vi "Initialize P40.vi"(8 "error in (no error)":errorcluster, 11 "SSI P40 Settings In":T1={"VISA resource name"="", "Simulated?"=TRUE}) -> (0 "error out":errorcluster, 1 "Initialized":bool, 2 "No Pump Connected":bool, 3 "SSI P40 Settings Out":T1={"VISA resource name"="", "Simulated?"=TRUE})   [LabVIEW 2021, in "SSI P40 Pump.lvlib"]
uses:
  SSI P40 Pump.lvlib
  SSI P40 Settings Cluster.ctl
  <vilib>/Instr/_visa.llb/VISA Configure Serial Port (Instr).vi
  <vilib>/regexp/Match Regular Expression.xnode
panel:
  out "read buffer 2":string
  out "read buffer":string
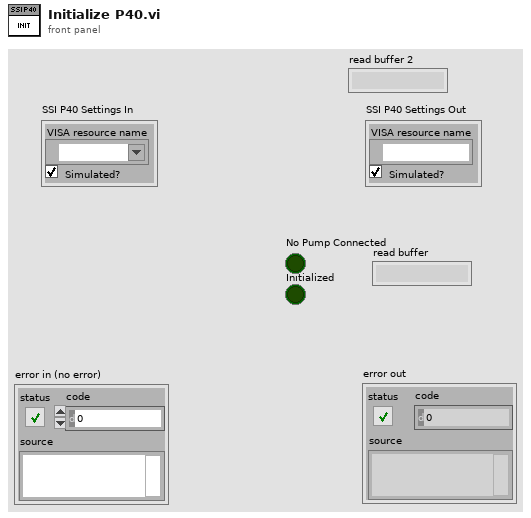
[diagram p1: front panel]
types:
  T1 = typedef "SSI P40 Pump.lvlib/SSI P40 Settings Cluster.ctl" = cluster{"VISA resource name":refnum<visa-resource-name>, "Simulated?":bool}
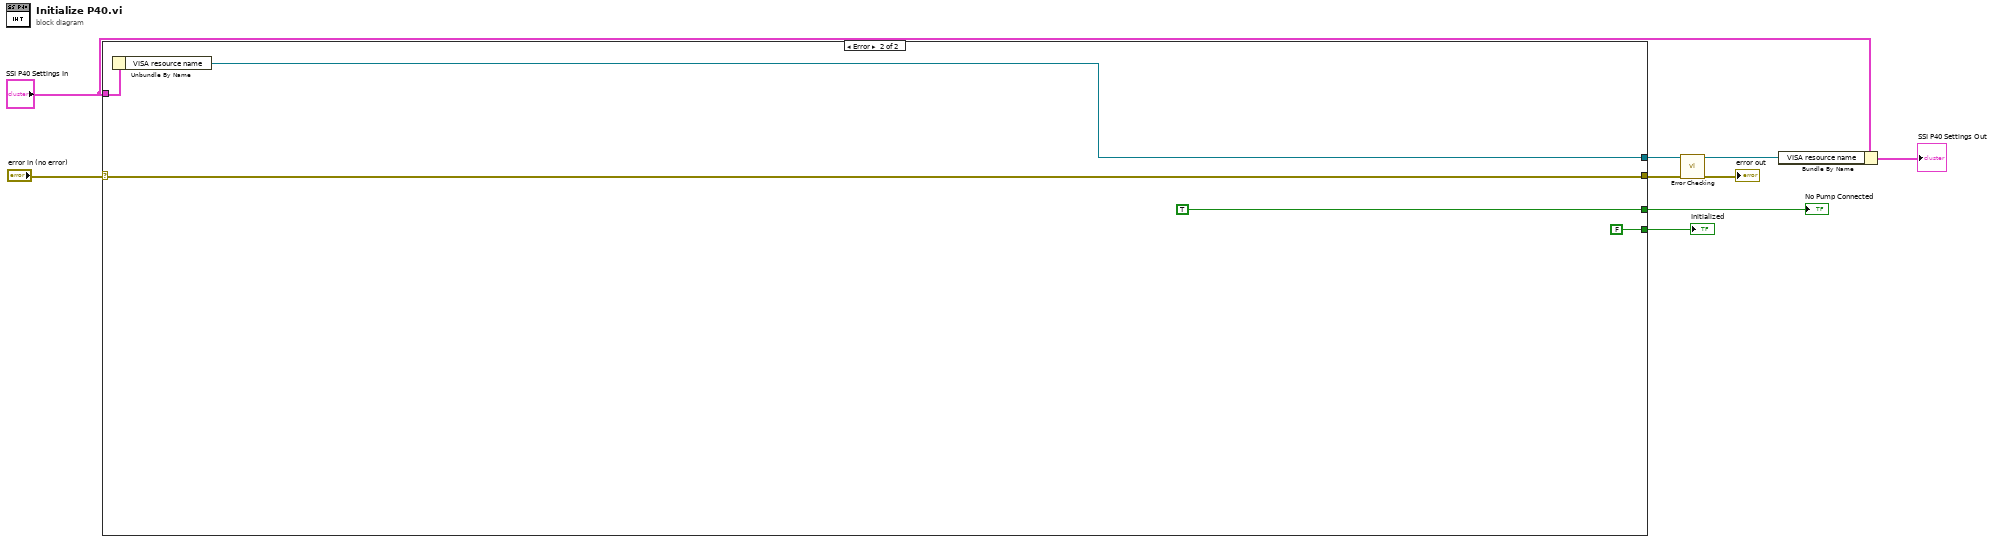
[diagram p0: block diagram]
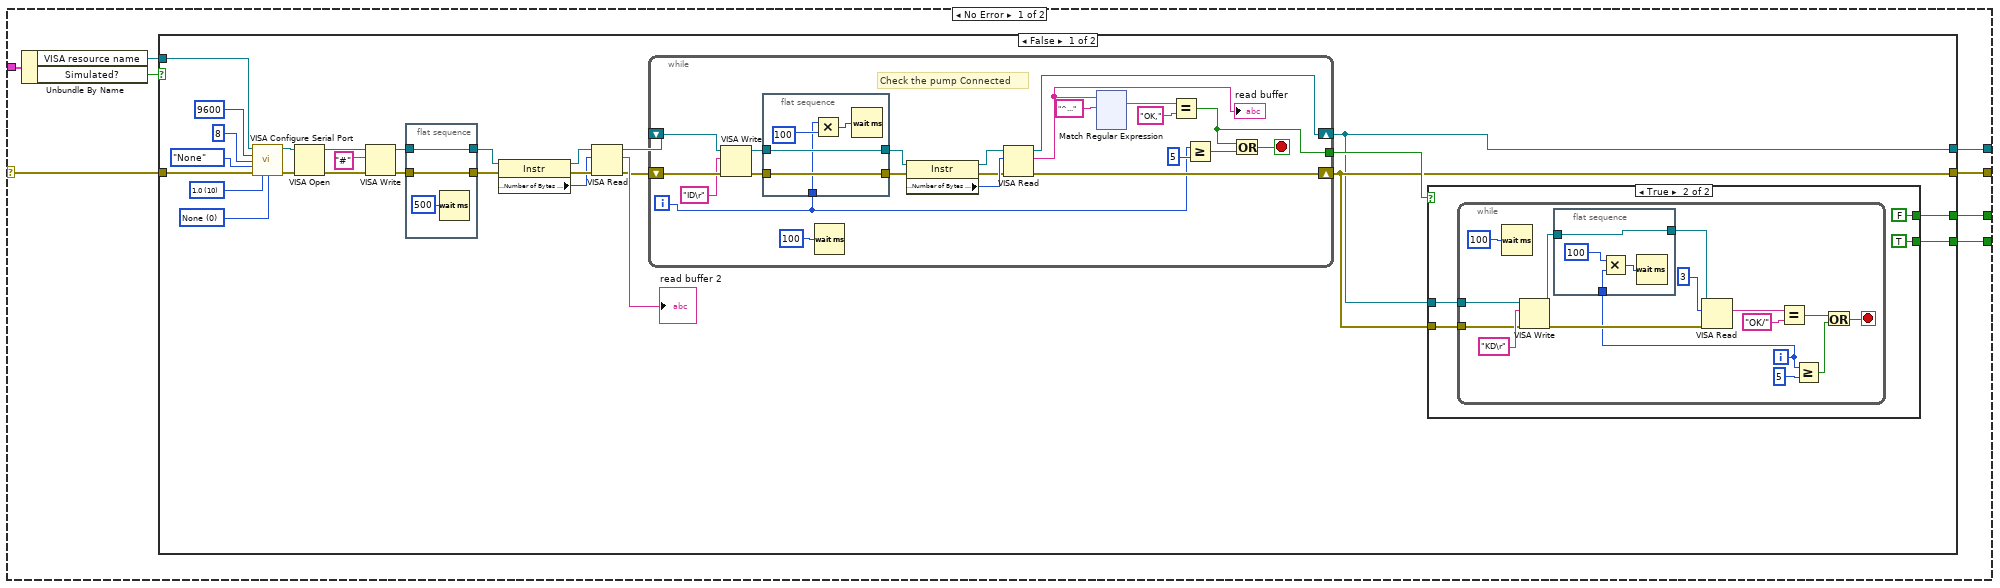
[diagram p2: hidden frame]
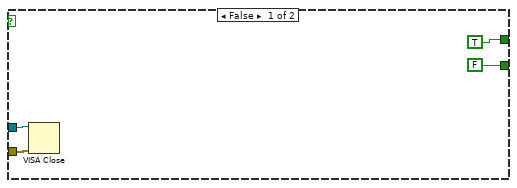
[diagram p3: hidden frame]
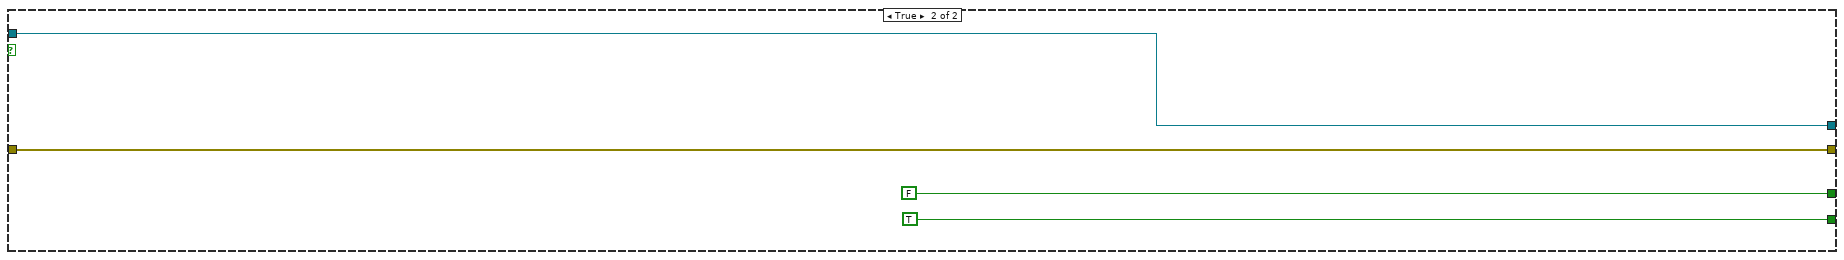
[diagram p4: hidden frame]
diagram:
  n1 = case shown="Error" "error in (no error)" {
    selector: "error in (no error)" -> [w17 w227]
    tunnel: "SSI P40 Settings In" -> [w13 w226]
    tunnel: [w14 w227] -> w6
    tunnel: [w12 w225] -> w5
    tunnel: [w11 FALSE] -> w4
    tunnel: [w10 TRUE] -> w3
    frame No Error {
      n2 = Unbundle By Name(w13) -> ("VISA resource name"=w15:refnum<visa-resource-name>, "Simulated?"=w16:bool)
      n3 = case shown="False" w16 {
        tunnel: w17 -> [w38 w222]
        tunnel: w15 -> [w36 w221]
        tunnel: [w32 w222] -> w14
        tunnel: [w31 w221] -> w12
        tunnel: [w30 TRUE] -> w11
        tunnel: [w18 FALSE] -> w10
        frame False {
          w40 = u16 0 items=["None", "XON/XOFF", "RTS/CTS", "XON/XOFF & RTS/CTS", "DTR/DSR", "XON/XOFF & DTR/DSR"] ("flow control (0:none)")
          w41 = u16 10 items=["1.0"=10, "1.5"=15, "2.0"=20] ("stop bits (10: 1 bit)")
          n4 = call-poly "VISA Configure Serial Port"("VISA resource name"=w36, "baud rate (9600)"=u32 9600, "data bits (8)"=u16 8, "parity (0:none)"=enum16{"None", "Odd", "Even", "Mark", "Space"}."None", "error in (no error)"=w38, "stop bits (10: 1 bit)"=w41, "flow control (0:none)"=w40) -> ("VISA resource name out"=w37:refnum<visa-resource-name>, "error out"=w39:errorcluster)  [unwired: 7 in]
          n5 = VISA Open(error in (no error)=w39, VISA resource name=w37) -> (VISA resource name=w35:refnum<visa-resource-name>, error out=w34:errorcluster)  [unwired: 3 in]
          n6 = VISA Write(VISA resource name=w35, write buffer="#", error in (no error)=w34) -> (VISA resource name out=w21:refnum<visa-resource-name>, error out=w19:errorcluster)  [unwired: 1 out]
          n7 = flat-sequence {
            tunnel: [w46] -> w22
            tunnel: w21 -> [w46]
            tunnel: [w45] -> w20
            tunnel: w19 -> [w45]
            frame #0 {
              n8 = Wait (ms)(milliseconds to wait=u32 500) -> ()  [unwired: 1 out]
            }
          }
          n9 = property class="Instr"(reference=w22, error in=w20) -> (reference out=w25:refnum<visa-resource-name>, error out=w26:errorcluster, "Serial Settings:Number of Bytes at Serial Port"=w24:u32)
          n10 = VISA Read(VISA resource name=w25, byte count=w24, error in (no error)=w26) -> (VISA resource name out=w27:refnum<visa-resource-name>, read buffer=→"read buffer 2":string, error out=w28:errorcluster)  [unwired: 1 out]
          n11 = while {
            tunnel: [w52] -> w33
            shift-right: [w68] -> w32
            shift-left: w28 -> [w60]
            shift-right: [w67] -> w31
            shift-left: w27 -> [w59]
            i -> [w48]
            stop <- w51 stop-if-true
            # "Check the pump Connected"
            n12 = VISA Write(VISA resource name=w59, write buffer="ID\r", error in (no error)=w60) -> (VISA resource name out=w56:refnum<visa-resource-name>, error out=w54:errorcluster)  [unwired: 1 out]
            n13 = flat-sequence {
              tunnel: [w74] -> w57
              tunnel: w56 -> [w74]
              tunnel: [w73] -> w55
              tunnel: w54 -> [w73]
              tunnel: w48 -> [w70]
              frame #0 {
                n14 = Multiply(x=w70, y=u32 100 ("milliseconds to wait")) -> (x*y=w72:u32)
                n15 = Wait (ms)(milliseconds to wait=w72) -> ()  [unwired: 1 out]
              }
            }
            n16 = Wait (ms)(milliseconds to wait=u32 100) -> ()  [unwired: 1 out]
            n17 = property class="Instr"(reference=w57, error in=w55) -> (reference out=w65:refnum<visa-resource-name>, error out=w64:errorcluster, "Serial Settings:Number of Bytes at Serial Port"=w66:u32)
            n18 = VISA Read(VISA resource name=w65, byte count=w66, error in (no error)=w64) -> (VISA resource name out=w67:refnum<visa-resource-name>, read buffer=w63:string, error out=w68:errorcluster)  [unwired: 1 out]
            "read buffer" <- w63
            n19 = xnode "Match Regular Expression"("input string"=w63, "regular expression"="^...") -> ("whole match"=w61:string)  [unwired: 4 in, 4 out]
            n20 = Equal?(x=w61, y="OK,") -> (x = y?=w52:bool)
            n21 = Greater Or Equal?(x=w48, y=5) -> (x >= y?=w53:bool)
            n22 = Or(x=w52, y=w53) -> (x .or. y?=w51:bool)
          }
          n23 = case shown="True" w33 {
            tunnel: w31 -> [w195 w197]
            tunnel: w32 -> [w194 w196]
            tunnel: [TRUE FALSE] -> w18
            tunnel: [FALSE TRUE] -> w30
            frame False {
              n24 = VISA Close(VISA resource name=w195, error in (no error)=w194) -> ()  [unwired: 1 out]
            }
            frame True {
              n25 = while {
                tunnel: w197 -> [w213]
                tunnel: w196 -> [w212]
                i -> [w200]
                stop <- w206 stop-if-true
                n26 = Wait (ms)(milliseconds to wait=u32 100) -> ()  [unwired: 1 out]
                n27 = VISA Write(VISA resource name=w213, write buffer="KD\r", error in (no error)=w212) -> (VISA resource name out=w202:refnum<visa-resource-name>, error out=w210:errorcluster)  [unwired: 1 out]
                n28 = flat-sequence {
                  tunnel: [w218] -> w201
                  tunnel: w202 -> [w218]
                  tunnel: w200 -> [w215]
                  frame #0 {
                    n29 = Multiply(x=u32 100 ("milliseconds to wait"), y=w215) -> (x*y=w217:u32)
                    n30 = Wait (ms)(milliseconds to wait=w217) -> ()  [unwired: 1 out]
                  }
                }
                n31 = VISA Read(VISA resource name=w201, byte count=u32 3, error in (no error)=w210) -> (read buffer=w209:string)  [unwired: 3 out]
                n32 = Equal?(x=w209, y="OK/") -> (x = y?=w207:bool)
                n33 = Greater Or Equal?(x=w200, y=5) -> (x >= y?=w204:bool)
                n34 = Or(x=w207, y=w204) -> (x .or. y?=w206:bool)
              }
            }
          }
        }
        frame True {
        }
      }
    }
    frame Error {
      n35 = Unbundle By Name(w226) -> ("VISA resource name"=w225:refnum<visa-resource-name>)
    }
  }
  "Initialized" <- w4
  "No Pump Connected" <- w3
  n36 = call "Error Checking.vi"("error in (no error)"=w6, "VISA resource name"=w5) -> ("error out"=→"error out":errorcluster, "VISA resource name"=w8:refnum<visa-resource-name>)  [unwired: 7 in, 1 out]
  n37 = Bundle By Name(cluster="SSI P40 Settings In", "VISA resource name"=w8) -> (→"SSI P40 Settings Out":T1)
